vi "error_out.vi"(8 "error in (no error)":errorcluster) -> (0 "error out":errorcluster)   [LabVIEW 2013, in "Experiment.lvclass"]
uses:
  Experiment.lvclass
  Globals.vi
  TCP_IP/TCP_IP.lvclass
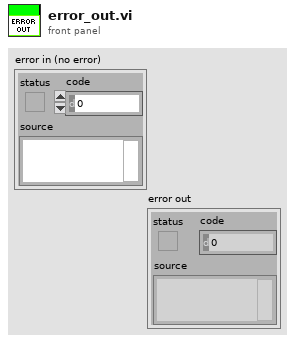
[diagram p1: front panel]
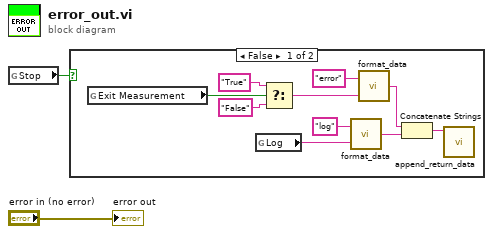
[diagram p0: block diagram]
diagram:
  n1 = global read "Globals.vi" "Stop"() -> (w2:bool)
  n2 = case shown="False" w2 {
    frame False {
      n3 = global read "Globals.vi" "Exit Measurement"() -> (w11:bool)
      n4 = global read "Globals.vi" "Log"() -> (w5:string)
      n5 = Select(t="True", s=w11, f="False") -> (s? t:f=w8:string)
      n6 = call "format_data.vi"("data"=w5, "name"="log") -> ("concatenated string"=w4:string)
      n7 = call "format_data.vi"("data"=w8, "name"="error") -> ("concatenated string"=w7:string)
      n8 = Concatenate Strings(w7, w4) -> (w3:string)
      n9 = call "append_return_data.vi"("Return Data"=w3) -> ()  [unwired: 11 in]
    }
    frame True {
    }
  }
  "error out" <- "error in (no error)"
